vi "Load RUS measurement.vi"(8 "error in (no error)":errorcluster, 11 "Common Measurements in":refnum<class "Common Measurements.lvclass">) -> (0 "error out":errorcluster, 3 "Common Measurements out":refnum<class "Common Measurements.lvclass">)   [LabVIEW 2015, in "Common Measurements.lvclass"]
uses:
  Common Measurements.lvclass
  Mag Lab Measure Base/Mag Lab Measure Base.lvclass
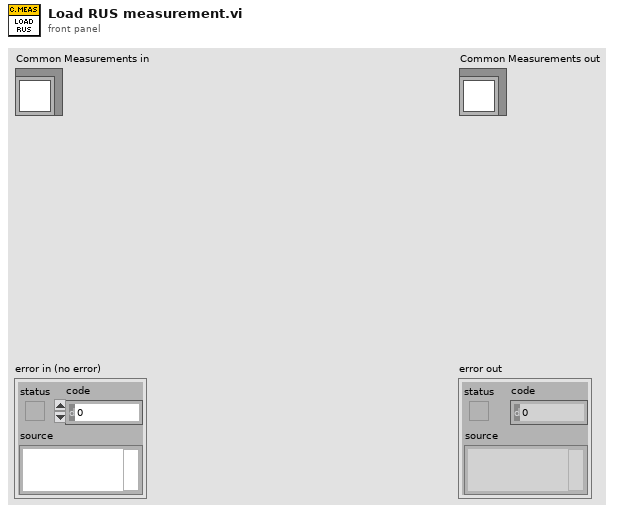
[diagram p1: front panel]
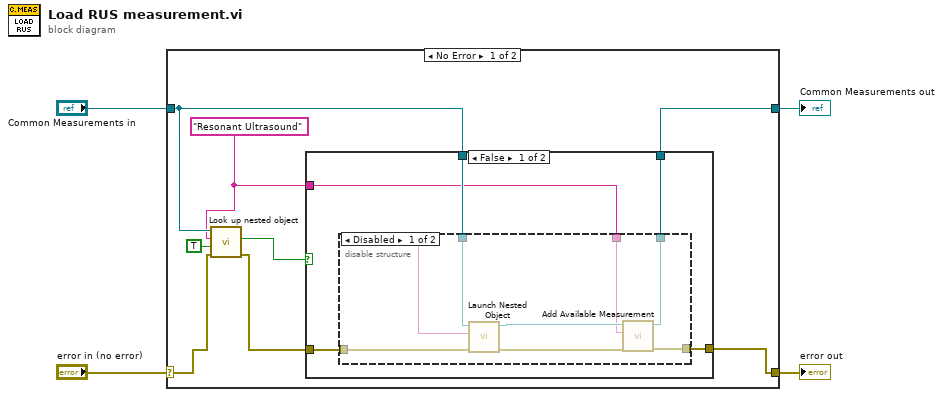
[diagram p0: block diagram]
diagram:
  n1 = case shown="No Error" "error in (no error)" {
    selector: "error in (no error)" -> [w8 w30]
    tunnel: [w12 w30] -> w3
    tunnel: [w11 w29] -> w1
    tunnel: "Common Measurements in" -> [w10 w29]
    frame No Error {
      w9 = "Resonant Ultrasound" ("Name")
      n2 = call "Look up nested object.vi"("error in (no error)"=w8, "Supress  dialog"=TRUE, "Object name"=w9, "Mag Lab Measure Base in"=w10) -> ("error out"=w7:errorcluster, "Found?"=w6:bool)  [unwired: 4 in, 2 out]
      n3 = case shown="False" w6 {
        tunnel: [w17 w28] -> w12
        tunnel: [w16 w27] -> w11
        tunnel: w10 -> [w15 w27]
        tunnel: w9 -> [w14 _]
        tunnel: w7 -> [w13 w28]
        frame False {
          n4 = disable-structure shown="Disabled" {
            disable-tunnel: [w23 w25] -> w17
            disable-tunnel: [w21 w26] -> w16
            disable-tunnel: w15 -> [w20 w26]
            disable-tunnel: w14 -> [w19 _]
            disable-tunnel: w13 -> [w18 w25]
            frame Disabled {
              n5 = call "Launch Nested Object.vi"("error in (no error)"=w18, "name"=w19, "Mag Lab Measure Base in"=w20) -> ("error out"=w24:errorcluster, "Mag Lab Measure Base out"=w22:refnum<class "Common Measurements.lvclass">)  [unwired: 6 in, 1 out]
              n6 = call-dynamic "Add Available Measurement.vi"("error in (no error)"=w24, "Name"=w19, "Common Measurements in"=w22) -> ("error out"=w23:errorcluster, "Common Measurements out"=w21:refnum<class "Common Measurements.lvclass">)  [unwired: 7 in]
            }
            frame Enabled {
            }
          }
        }
        frame True {
        }
      }
    }
    frame Error {
    }
  }
  "error out" <- w3
  "Common Measurements out" <- w1
